vi "Clot.vi"() -> ()   [LabVIEW 2022 SP3]
uses:
  <vilib>/Motion/FlexMotion/CustomControls/CustomControls.llb/AxisOrVectorSpace To Configure.flx
  <vilib>/Motion/FlexMotion/FunctionsVIs/StartStopMotion.llb/Stop Motion (8 axes).flx
panel:
  out "Custom Wave":waveform(i16)(graph)
  out "Actual Time":sgl format="%.2f"
  out "Progress":dbl(slide) scale=0.0..1.0 scale format="%.2f"
  in  "Panametrics":bool
  in  "Temp":bool=TRUE
  in  "Motion Stage Type":u16(ring)=2 items=["MM 2000", "Servo", "Stepper"]
  in  "Digitizer":bool
  in  "Move Motors":bool
  in  "START EXP":bool
  in  "QUIT":bool
  out "Current Pass":i32
  in  "Exp Select":enum32{"PW", "Stop and Go", "F Balance"}(tab)
  out "Length time (s)":sgl=1.0 min=-2e+07 max=2e+07 format="%.2f"
  out "Number of passes":i32
  in  "exp per cycle  (ms)":sgl=0.5 format="%.3f"
  in  "scan length (cm)":sgl=1.0 min=-2e+07 max=2e+07 format="%.2f"
  in  "Total exp time (s)":dbl=10.0 format="%.2f"
  in  "Velocity (cm/s)":sgl=1.0 format="%.2f"
  in  "duty cycle":dbl=0.5 format="%.3f"
  out "PRF (Hz)":dbl=1000.0
  in  "Load Wave?":bool
  in  "2nd Busrt Scale":dbl=0.5
  in  "Mode":bool caption="Boolean"
  in  "Exp time (s)":dbl=0.3 format="%.2f"
  in  "exp per cycle  (ms) sg":sgl=0.5 format="%.3f"
  in  "duty cycle sq":dbl=0.5 caption="duty cycle sg" format="%.3f"
  out "PRF (Hz) sg":dbl=1000.0 caption="PRF (Hz)"
  out "Total exp pts":i16=1
  out "Total one way dist (mm)":sgl=1.0 format="%.2f"
  in  "Number of Repeats":i16=1
  in  "Total exp pts in one direction":i16=2 min=2
  in  "Time for move between exp (s)":sgl=1.0 format="%.2f"
  in  "Dist between exp (mm)":sgl=1.0 format="%.2f"
  in  "On time (s)":dbl=0.3 format="%.2f"
  # "Motion system is initialized on first execution. Wait for motion window to open before turning on motor amplifier. Function generator must be in burst, ext gate mode. The Ext Trig on grey box goes to gate of HP 3352A. Stages return to start position after scan or if scan interupted. TURN OFF ENI BEFORE QUITING LABVIEW!"
  # "Red means off, green means active. Scan can be stopped by switching to red."
  # "Motion may stop mid length if actual time exceeds Total exp time."
  # "Exposure Values"
  # "Motion values"
  # "Exposure Values"
  # "Pressing Start Exp turns on  therapy device for specified on time."
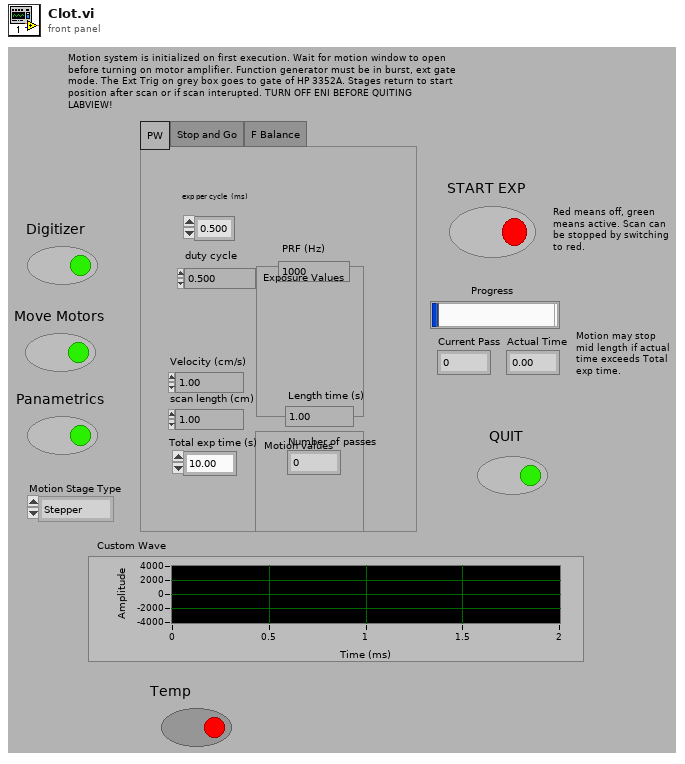
[diagram p1: front panel]
types:
  T1 = typedef "AxisOrVectorSpace To Configure.flx" = u16
  T2 = enum16{"Absolute Position", "Relative Position", "Velocity", "Relative to Cap Pos", "Modulus Position", "Absolute Contouring", "Relative Contouring"}
  T3 = typedef "Resource Out (Enum).flx" = u16
  T4 = typedef "Bd Id Out" = u8
  T5 = cluster{"Reserved":bool, "Axis #1 Move Complete":bool, "Axis #2 Move Complete":bool, "Axis #3 Move Complete":bool, "Axis #4 Move Complete":bool, "Axis #5 Move Complete":bool, "Axis #6 Move Complete":bool, "Axis #7 Move Complete":bool, "Axis #8 Move Complete":bool, "Axis #9 MoveComplete":bool, "Axis #10 Move Complete":bool, "Axis #11 Move Complete":bool, "Axis #12 Move Complete":bool, "Status #13":bool, "Status #14":bool, "Status #15":bool}
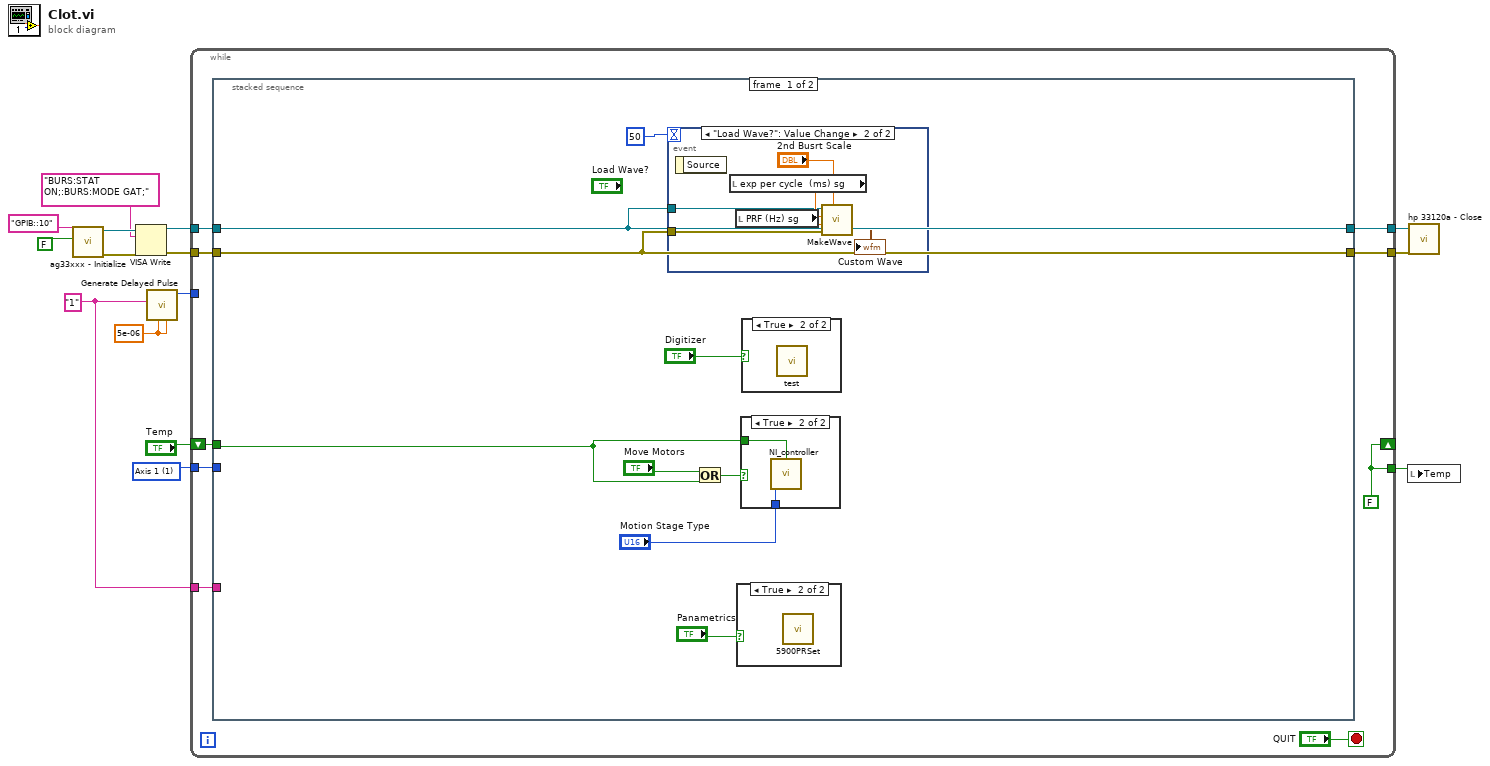
[diagram p0: block diagram]
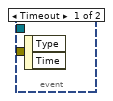
[diagram p2: hidden frame]
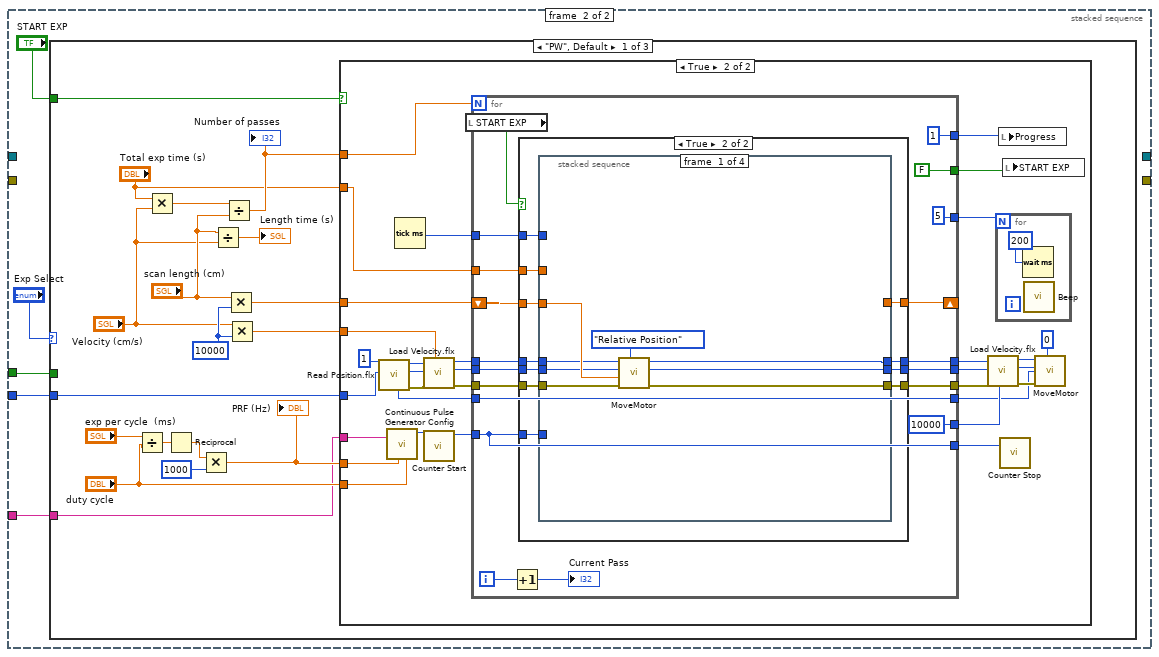
[diagram p6: hidden frame]
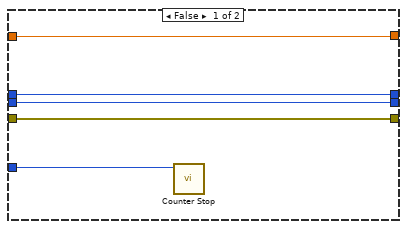
[diagram p8: hidden frame]
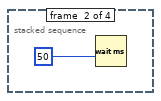
[diagram p9: hidden frame]
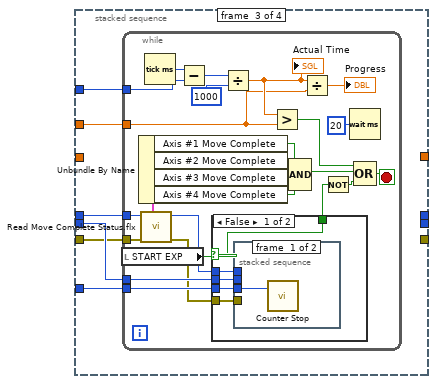
[diagram p10: hidden frame]
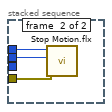
[diagram p11: hidden frame]
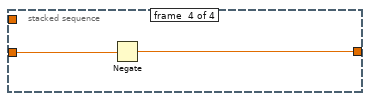
[diagram p13: hidden frame]
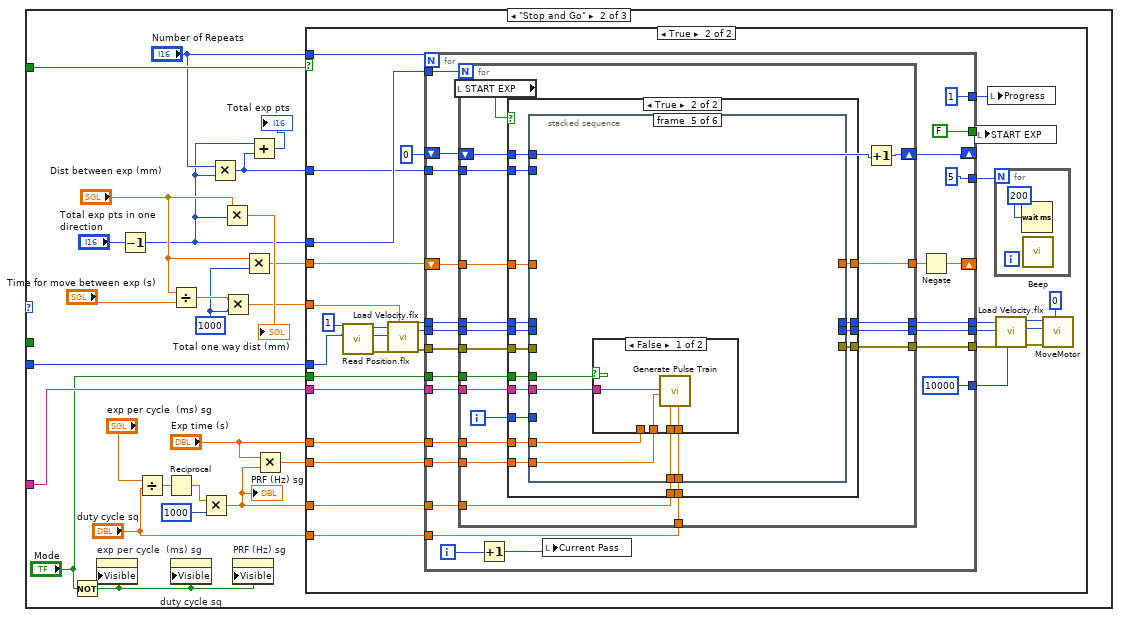
[diagram p14: hidden frame]
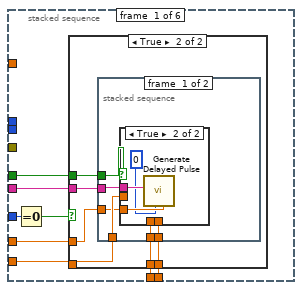
[diagram p17: hidden frame]
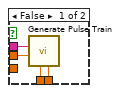
[diagram p19: hidden frame]
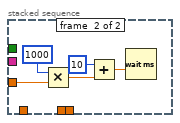
[diagram p20: hidden frame]
diagram:
  w10 = T1 1 items=["Axis 1"=1, "Axis 2"=2, "Axis 3"=3, "Axis 4"=4, "Axis 5"=5, "Axis 6"=6, "Vector Space 1"=17, "Vector Space 2"=18, "Vector Space 3"=19] ("Axis or Vector Space")
  w11 = "1"
  w13 = 5e-06
  n1 = call <instrlib>:"ag33xxx - Initialize.vi"("ID Query (T: Check)"=FALSE, "Instrument Resource Name"="GPIB::10" ("HP33120A Burst")) -> ("error out"=w7:errorcluster, "dup VISA session"=w8:refnum<visa-resource-name>)  [unwired: 8 in]
  n2 = VISA Write(VISA resource name=w8, write buffer="BURS:STAT ON;:BURS:MODE GAT;", error in (no error)=w7) -> (VISA resource name out=w5:refnum<visa-resource-name>, error out=w4:errorcluster)  [unwired: 1 out]
  n3 = call <vilib>:"Generate Delayed Pulse.vi"("pulse width (s or cycles)"=w13, "pulse delay (s or cycles)"=w13, "counter"=w11) -> ("[taskID]"=w12:u32)  [unwired: 6 in, 2 out]
  n4 = while {
    shift-right: [w22] -> _
    shift-left: "Temp" -> [w23]
    tunnel: [w22] -> w14
    tunnel: w12 -> [_]
    tunnel: w11 -> [w21]
    tunnel: w10 -> [w20]
    tunnel: w5 -> [w19]
    tunnel: w4 -> [w18]
    tunnel: [w17] -> w3
    tunnel: [w16] -> w2
    stop <- "QUIT" stop-if-true
    w22 = FALSE
    n5 = stacked-sequence {
      tunnel: w23 -> [w28 w46]
      tunnel: w21 -> [_ w44]
      tunnel: w20 -> [_ w43]
      tunnel: w19 -> [w26 _]
      tunnel: w18 -> [w25 _]
      tunnel: [w26 _] -> w17
      tunnel: [w25 _] -> w16
      frame #0 {
        n6 = event shown="[1] \"Load Wave?\": Value Change" {
          selector: _ -> [_ _]
          dyn-events: _ -> [_ _]
          timeout: 50 -> [_ _]
          tunnel: w26 -> [_ w36]
          tunnel: w25 -> [_ w35]
          event Timeout {
            n7 = event-data() -> ()  [unwired: 1 in, 2 out]
          }
          event "Load Wave?": Value Change {
            n8 = event-data() -> ()  [unwired: 1 in, 1 out]
            n9 = local read "exp per cycle  (ms) sg"() -> (w38:sgl)
            n10 = local read "PRF (Hz) sg"() -> (w39:dbl)
            n11 = call "MakeWave.vi"("Instrument Resource Name"=w36, "exp per cycle  (ms) sg"=w38, "PRF (Hz) sg"=w39, "error in (no error)"=w35, "2nd Busrt Scale"="2nd Busrt Scale") -> ("output waveform"=→"Custom Wave":waveform(i16))  [unwired: 1 out]
          }
        }
        n12 = Or(x="Move Motors", y=w28) -> (x .or. y?=w29:bool)
        n13 = case shown="True" "Panametrics" {
          frame False {
          }
          frame True {
            n14 = call "5900PRSet.vi"() -> ()  [unwired: 13 in, 3 out]
          }
        }
        n15 = case shown="True" w29 {
          tunnel: "Motion Stage Type" -> [_ w41]
          tunnel: w28 -> [_ w40]
          frame False {
          }
          frame True {
            n16 = call "NI_controller.VI"("Initialize"=w40, "Motion System"=w41) -> ()  [unwired: 3 in, 1 out]
          }
        }
        n17 = case shown="True" "Digitizer" {
          frame False {
          }
          frame True {
            n18 = call "test.vi"() -> ()  [unwired: 4 in, 4 out]
          }
        }
      }
      frame #1 {
        n19 = case shown="\"PW\", Default" "Exp Select" {
          tunnel: w46 -> [_ _ _]
          tunnel: w44 -> [w49 w203 w393]
          tunnel: w43 -> [w48 w204 _]
          tunnel: "START EXP" -> [w47 w208 w395]
          frame "PW", Default {
            w64 = 10000
            n20 = Divide(x="exp per cycle  (ms)", y="duty cycle") -> (x/y=w61:dbl)
            n21 = Multiply(x="Total exp time (s)", y="Velocity (cm/s)") -> (x*y=w63:dbl)
            n22 = Reciprocal(x=w61) -> (1/x=w60:dbl)
            n23 = Multiply(x=w60, y=1000) -> (x*y=w55:dbl)
            "PRF (Hz)" <- w55
            n24 = Divide(x="scan length (cm)", y="Velocity (cm/s)") -> (x/y=→"Length time (s)":sgl)
            n25 = Divide(x=w63, y="scan length (cm)") -> (x/y=w56:dbl)
            "Number of passes" <- w56
            n26 = Multiply(x="scan length (cm)", y=w64) -> (x*y=w58:sgl)
            n27 = Multiply(x="Velocity (cm/s)", y=w64) -> (x*y=w57:sgl)
            n28 = case shown="True" w47 {
              tunnel: w58 -> [_ w93]
              tunnel: w57 -> [_ w92]
              tunnel: w56 -> [_ w91]
              tunnel: w55 -> [_ w90]
              tunnel: "duty cycle" -> [_ w89]
              tunnel: "Total exp time (s)" -> [_ w85]
              tunnel: w49 -> [_ w66]
              tunnel: w48 -> [_ w65]
              frame False {
              }
              frame True {
                n29 = call <vilib>:"Read Position.flx"("Axis"=w65, "Board ID"=1) -> ("error out"=w80:errorcluster, "Resource Output"=w79:T3, "Bd ID Out"=w82:T4, "Position"=w72:i32)  [unwired: 4 in]
                n30 = call <vilib>:"Continuous Pulse Generator Config.vi"("duty cycle (0.5)"=w89, "frequency (Hz)"=w90, "counter"=w66) -> ("taskID"=w96:u32)  [unwired: 5 in, 3 out]
                n31 = Tick Count (ms)() -> (millisecond timer value=w84:u32)
                n32 = call <vilib>:"Load Velocity.flx"("Velocity (10000)"=w92, "error in (no error)"=w80, "Axis or Vector Space"=w79, "Board ID"=w82) -> ("error out"=w74:errorcluster, "Resource Output"=w78:T3, "Bd ID Out"=w77:T4)  [unwired: 3 in]
                n33 = call <vilib>:"Counter Start.vi"("taskID"=w96) -> ("taskID"=w95:u32)  [unwired: 9 in, 1 out]
                n34 = for {
                  N: w91 -> [_]
                  shift-right: [w114] -> _
                  shift-left: w93 -> [w116]
                  tunnel: w77 -> [w115]
                  tunnel: w95 -> [w113]
                  tunnel: [w113] -> w94
                  tunnel: [FALSE] -> w86
                  tunnel: [5] -> w88
                  tunnel: [10000] -> w87
                  tunnel: w85 -> [w106]
                  tunnel: w84 -> [w105]
                  tunnel: [1] -> w83
                  tunnel: w78 -> [w103]
                  tunnel: [w102] -> w76
                  tunnel: [w101] -> w75
                  tunnel: w74 -> [w100]
                  tunnel: [w99] -> w73
                  tunnel: [w98] -> w68
                  tunnel: w72 -> [w98]
                  i -> [w111]
                  n35 = local read "START EXP"() -> (w107:bool)
                  n36 = Increment(x=w111) -> (x+1=→"Current Pass":i32)
                  n37 = case shown="True" w107 {
                    tunnel: w116 -> [w120 w132]
                    tunnel: w115 -> [w119 w131]
                    tunnel: [w120 w130] -> w114
                    tunnel: w113 -> [w121 w129]
                    tunnel: w106 -> [_ w128]
                    tunnel: w105 -> [_ w127]
                    tunnel: w103 -> [w118 w126]
                    tunnel: [w119 w125] -> w102
                    tunnel: [w118 w124] -> w101
                    tunnel: w100 -> [w117 w123]
                    tunnel: [w117 w122] -> w99
                    frame False {
                      n38 = call <vilib>:"Counter Stop.vi"("taskID"=w121) -> ()  [unwired: 5 in, 2 out]
                    }
                    frame True {
                      n39 = stacked-sequence {
                        tunnel: w132 -> [w140 _ _ w184]
                        tunnel: w131 -> [w136 _ w147 _]
                        tunnel: [_ _ _ w183] -> w130
                        tunnel: w129 -> [_ _ w146 _]
                        tunnel: w128 -> [_ _ w145 _]
                        tunnel: w127 -> [_ _ w144 _]
                        tunnel: w126 -> [w133 _ w143 _]
                        tunnel: [w135 _ _ _] -> w125
                        tunnel: [w134 _ _ _] -> w124
                        tunnel: w123 -> [w138 _ w142 _]
                        tunnel: [w137 _ _ _] -> w122
                        frame #0 {
                          n40 = call "MoveMotor.vi"("Position Mode (Absolute)"=T2."Relative Position", "error in (no error)"=w138, "Target Position (0)"=w140, "Axis or Vector Space"=w133, "Motion Bd ID"=w136) -> ("error out"=w137:errorcluster, "Resource Output"=w134:u16, "Bd ID Out"=w135:u8)  [unwired: 4 in]
                        }
                        frame #1 {
                          n41 = Wait (ms)(milliseconds to wait=50) -> ()  [unwired: 1 out]
                        }
                        frame #2 {
                          n42 = while {
                            tunnel: w147 -> [w167]
                            tunnel: w146 -> [w165]
                            tunnel: w143 -> [w164]
                            tunnel: w145 -> [w149]
                            tunnel: w144 -> [w155]
                            tunnel: w142 -> [w152]
                            stop <- w161 stop-if-true
                            n43 = local read "START EXP"() -> (w166:bool)
                            n44 = call <vilib>:"Read Move Complete Status.flx"("error in (no error)"=w152, "Board ID"=w167) -> ("error out"=w151:errorcluster, "Bd ID Out"=w153:T4, "Move Complete Status"=w172:T5)  [unwired: 4 in]
                            n45 = Unbundle By Name(w172) -> ("Axis #1 Move Complete"=w171:bool, "Axis #2 Move Complete"=w170:bool, "Axis #3 Move Complete"=w169:bool, "Axis #4 Move Complete"=w168:bool)
                            n46 = Tick Count (ms)() -> (millisecond timer value=w160:u32)
                            n47 = Subtract(x=w160, y=w155) -> (x-y=w159:u32)
                            n48 = case shown="False" w166 {
                              selector: w166 -> [w174 w182]
                              tunnel: w165 -> [w177 _]
                              tunnel: w164 -> [w176 _]
                              tunnel: w153 -> [w175 _]
                              tunnel: [w174 w182] -> w162
                              tunnel: w151 -> [w173 _]
                              frame False {
                                n49 = stacked-sequence {
                                tunnel: w177 -> [w178 _]
                                tunnel: w176 -> [_ w181]
                                tunnel: w175 -> [_ w180]
                                tunnel: w173 -> [_ w179]
                                frame #0 {
                                n50 = call <vilib>:"Counter Stop.vi"("taskID"=w178) -> ()  [unwired: 5 in, 2 out]
                                }
                                frame #1 {
                                n51 = call-poly <vilib>:"Stop Motion.flx"("error in (no error)"=w179, "Axis or Vector Space"=w181, "Board ID"=w180) -> ()  [unwired: 4 in, 3 out]
                                }
                                }
                              }
                              frame True {
                              }
                            }
                            n52 = Divide(x=w159, y=1000) -> (x/y=w150:dbl)
                            "Actual Time" <- w150
                            n53 = Greater?(x=w150, y=w149) -> (0:w148:bool)
                            n54 = Compound Arithmetic op=AND(w171, w170, w169, w168) -> (w163:bool)
                            n55 = Divide(x=w150, y=w149) -> (x/y=→"Progress":dbl)
                            n56 = Not(x=w162) -> (.not. x?=w154:bool)
                            n57 = Wait (ms)(milliseconds to wait=20) -> ()  [unwired: 1 out]
                            n58 = Compound Arithmetic op=OR(w148, w163, w154) -> (w161:bool)
                          }
                        }
                        frame #3 {
                          n59 = Negate(x=w184) -> (-x=w183:sgl)
                        }
                      }
                    }
                  }
                }
                n60 = call <vilib>:"Load Velocity.flx"("Velocity (10000)"=w87, "error in (no error)"=w73, "Axis or Vector Space"=w75, "Board ID"=w76) -> ("error out"=w70:errorcluster, "Resource Output"=w69:T3, "Bd ID Out"=w71:T4)  [unwired: 3 in]
                n61 = for {
                  N: w88 -> [_]
                  n62 = Wait (ms)(milliseconds to wait=200) -> ()  [unwired: 1 out]
                  n63 = call <vilib>:"Beep.vi"() -> ()  [unwired: 12 in]
                }
                n64 = local write "Progress"(w83) -> ()
                n65 = call <vilib>:"Counter Stop.vi"("taskID"=w94) -> ()  [unwired: 5 in, 2 out]
                n66 = local write "START EXP"(w86) -> ()
                n67 = call "MoveMotor.vi"("Position Mode (Absolute)"=0, "error in (no error)"=w70, "Target Position (0)"=w68, "Axis or Vector Space"=w69, "Motion Bd ID"=w71) -> ()  [unwired: 4 in, 3 out]
              }
            }
          }
          frame "Stop and Go" {
            w201 = 1000
            n68 = Not(x="Mode") -> (.not. x?=w188:bool)
            n69 = property on="exp per cycle  (ms) sg" class="DigNum (strict)"("Visible"=w188) -> ()  [unwired: 2 in, 2 out]
            n70 = Decrement(x="Total exp pts in one direction") -> (x-1=w185:i16)
            n71 = Divide(x="exp per cycle  (ms) sg", y="duty cycle sq") -> (x/y=w197:dbl)
            n72 = Reciprocal(x=w197) -> (1/x=w196:dbl)
            n73 = Divide(x="Dist between exp (mm)", y="Time for move between exp (s)") -> (x/y=w206:sgl)
            n74 = property on="duty cycle sq" class="DigNum (strict)"("Visible"=w188) -> ()  [unwired: 2 in, 2 out]
            n75 = Multiply(x=w196, y=1000) -> (x*y=w191:dbl)
            "PRF (Hz) sg" <- w191
            n76 = Multiply(x="Number of Repeats", y=w185) -> (x*y=w187:i16)
            n77 = Multiply(x="Dist between exp (mm)", y=w185) -> (x*y=→"Total one way dist (mm)":sgl)
            n78 = Multiply(x=w206, y=w201) -> (x*y=w205:sgl)
            n79 = property on="PRF (Hz) sg" class="DigNum (strict)"("Visible"=w188) -> ()  [unwired: 2 in, 2 out]
            n80 = Multiply(x="Dist between exp (mm)", y=w201) -> (x*y=w200:sgl)
            n81 = Add(x=w185, y=w187) -> (x+y=→"Total exp pts":i16)
            n82 = Multiply(x="Exp time (s)", y=w191) -> (x*y=w190:dbl)
            n83 = case shown="True" w208 {
              tunnel: w205 -> [_ w232]
              tunnel: w204 -> [_ w231]
              tunnel: w203 -> [_ w222]
              tunnel: "Exp time (s)" -> [_ w221]
              tunnel: "Number of Repeats" -> [_ w220]
              tunnel: w200 -> [_ w219]
              tunnel: w185 -> [_ w216]
              tunnel: w187 -> [_ w215]
              tunnel: "duty cycle sq" -> [_ w213]
              tunnel: w191 -> [_ w212]
              tunnel: w190 -> [_ w211]
              tunnel: "Mode" -> [_ w210]
              frame False {
              }
              frame True {
                n84 = call <vilib>:"Read Position.flx"("Axis"=w231, "Board ID"=1) -> ("error out"=w238:errorcluster, "Resource Output"=w237:T3, "Bd ID Out"=w240:T4)  [unwired: 4 in, 1 out]
                n85 = call <vilib>:"Load Velocity.flx"("Velocity (10000)"=w232, "error in (no error)"=w238, "Axis or Vector Space"=w237, "Board ID"=w240) -> ("error out"=w228:errorcluster, "Resource Output"=w229:T3, "Bd ID Out"=w230:T4)  [unwired: 3 in]
                n86 = for {
                  N: w220 -> [_]
                  shift-right: [w251] -> _
                  shift-left: w219 -> [w265]
                  tunnel: [FALSE] -> w217
                  tunnel: [5] -> w227
                  tunnel: [10000] -> w223
                  tunnel: [1] -> w218
                  tunnel: [w259] -> w226
                  tunnel: [w258] -> w225
                  tunnel: [w257] -> w224
                  tunnel: w230 -> [w256]
                  tunnel: w229 -> [w255]
                  tunnel: w228 -> [w254]
                  tunnel: w222 -> [w253]
                  tunnel: w221 -> [w252]
                  tunnel: w216 -> [w250]
                  tunnel: w215 -> [w249]
                  shift-right: [w247] -> _
                  shift-left: 0 -> [w248]
                  tunnel: w213 -> [w246]
                  tunnel: w212 -> [w245]
                  tunnel: w211 -> [w244]
                  tunnel: w210 -> [w243]
                  i -> [w242]
                  n87 = for {
                    N: w250 -> [_]
                    tunnel: w265 -> [w284]
                    tunnel: [w283] -> w264
                    tunnel: [w281] -> w259
                    tunnel: [w280] -> w258
                    tunnel: [w279] -> w257
                    tunnel: w256 -> [w278]
                    tunnel: w255 -> [w277]
                    tunnel: w254 -> [w276]
                    tunnel: w253 -> [w275]
                    tunnel: w252 -> [w274]
                    tunnel: w249 -> [w272]
                    shift-right: [w271] -> w247
                    shift-left: w248 -> [w270]
                    tunnel: w246 -> [w269]
                    tunnel: w245 -> [w268]
                    tunnel: w244 -> [w267]
                    tunnel: w243 -> [w266]
                    i -> [w273]
                    n88 = local read "START EXP"() -> (w282:bool)
                    n89 = case shown="True" w282 {
                      tunnel: w284 -> [w288 w305]
                      tunnel: [w288 w304] -> w283
                      tunnel: [w287 w303] -> w281
                      tunnel: [w286 w302] -> w280
                      tunnel: [w285 w301] -> w279
                      tunnel: w278 -> [w287 w298]
                      tunnel: w277 -> [w286 w297]
                      tunnel: w276 -> [w285 w296]
                      tunnel: w275 -> [_ w300]
                      tunnel: w274 -> [_ w299]
                      tunnel: w273 -> [_ w295]
                      tunnel: w272 -> [_ w294]
                      tunnel: w270 -> [_ w293]
                      tunnel: w269 -> [_ w292]
                      tunnel: w268 -> [_ w291]
                      tunnel: w267 -> [_ w290]
                      tunnel: w266 -> [_ w289]
                      frame False {
                      }
                      frame True {
                        n90 = stacked-sequence {
                          tunnel: w305 -> [_ w345 _ _ _ w391]
                          tunnel: [_ _ _ _ _ w391] -> w304
                          tunnel: [_ w342 _ _ _ _] -> w303
                          tunnel: [_ w341 _ _ _ _] -> w302
                          tunnel: [_ w343 _ _ _ _] -> w301
                          tunnel: w300 -> [w313 _ _ _ w375 _]
                          tunnel: w299 -> [w312 _ _ _ w373 w386]
                          tunnel: w298 -> [_ w340 _ w350 _ _]
                          tunnel: w297 -> [_ w339 _ _ _ _]
                          tunnel: w296 -> [_ w338 _ w349 _ _]
                          tunnel: w295 -> [w311 _ _ _ _ _]
                          tunnel: w294 -> [_ _ _ w348 _ _]
                          tunnel: w293 -> [_ _ _ w347 _ _]
                          tunnel: w292 -> [w309 _ _ _ w378 _]
                          tunnel: w291 -> [w308 _ _ _ w377 _]
                          tunnel: w290 -> [w307 _ _ _ w376 _]
                          tunnel: w289 -> [w306 _ _ _ w374 _]
                          frame #0 {
                            n91 = Equal To 0?(x=w311) -> (x = 0?=w310:bool)
                            n92 = case shown="True" w310 {
                              tunnel: w313 -> [_ w319]
                              tunnel: w312 -> [_ w315]
                              tunnel: w309 -> [_ w318]
                              tunnel: w308 -> [_ w317]
                              tunnel: w307 -> [_ w316]
                              tunnel: w306 -> [_ w314]
                              frame False {
                              }
                              frame True {
                                n93 = stacked-sequence {
                                tunnel: w319 -> [w323 _]
                                tunnel: w318 -> [w325 _]
                                tunnel: w317 -> [w324 _]
                                tunnel: w316 -> [w322 _]
                                tunnel: w315 -> [w320 w333]
                                tunnel: w314 -> [w321 _]
                                frame #0 {
                                n94 = case shown="True" w321 {
                                tunnel: w325 -> [w329 _]
                                tunnel: w324 -> [w328 _]
                                tunnel: w323 -> [w327 w332]
                                tunnel: w322 -> [w326 _]
                                tunnel: w320 -> [_ w331]
                                frame False {
                                n95 = call <vilib>:"Generate Pulse Train.vi"("duty cycle (0.5)"=w329, "frequency (Hz)"=w328, "number of pulses (cont:0)"=w326, "counter"=w327) -> ()  [unwired: 5 in, 3 out]
                                }
                                frame True {
                                n96 = call <vilib>:"Generate Delayed Pulse.vi"("pulse width (s or cycles)"=w331, "pulse delay (s or cycles)"=0, "counter"=w332) -> ()  [unwired: 6 in, 3 out]
                                }
                                }
                                }
                                frame #1 {
                                n97 = Multiply(x=1000, y=w333) -> (x*y=w335:dbl)
                                n98 = Add(x=10, y=w335) -> (x+y=w336:dbl)
                                n99 = Wait (ms)(milliseconds to wait=w336) -> ()  [unwired: 1 out]
                                }
                                }
                              }
                            }
                          }
                          frame #1 {
                            n100 = call "MoveMotor.vi"("Position Mode (Absolute)"=T2."Relative Position", "error in (no error)"=w338, "Target Position (0)"=w345, "Axis or Vector Space"=w339, "Motion Bd ID"=w340) -> ("error out"=w343:errorcluster, "Resource Output"=w341:u16, "Bd ID Out"=w342:u8)  [unwired: 4 in]
                          }
                          frame #2 {
                            n101 = Wait (ms)(milliseconds to wait=50) -> ()  [unwired: 1 out]
                          }
                          frame #3 {
                            n102 = while {
                              tunnel: w350 -> [w354]
                              tunnel: w349 -> [w353]
                              tunnel: w348 -> [w352]
                              tunnel: w347 -> [w351]
                              stop <- w360 stop-if-true
                              n103 = local read "START EXP"() -> (w363:bool)
                              n104 = call <vilib>:"Read Move Complete Status.flx"("error in (no error)"=w353, "Board ID"=w354) -> ("error out"=w356:errorcluster, "Bd ID Out"=w357:T4, "Move Complete Status"=w368:T5)  [unwired: 4 in]
                              n105 = Unbundle By Name(w368) -> ("Axis #1 Move Complete"=w367:bool, "Axis #2 Move Complete"=w366:bool, "Axis #3 Move Complete"=w365:bool, "Axis #4 Move Complete"=w364:bool)
                              n106 = case shown="False" w363 {
                                selector: w363 -> [w370 w372]
                                tunnel: w357 -> [w371 _]
                                tunnel: [w370 w372] -> w361
                                tunnel: w356 -> [w369 _]
                                frame False {
                                n107 = call-poly <vilib>:"Stop Motion.flx"("error in (no error)"=w369, "Board ID"=w371) -> ()  [unwired: 5 in, 3 out]
                                }
                                frame True {
                                }
                              }
                              n108 = Divide(x=w351, y=w352) -> (x/y=w355:dbl)
                              n109 = local write "Progress"(w355) -> ()
                              n110 = Compound Arithmetic op=AND(w367, w366, w365, w364) -> (w362:bool)
                              n111 = Not(x=w361) -> (.not. x?=w358:bool)
                              n112 = Wait (ms)(milliseconds to wait=20) -> ()  [unwired: 1 out]
                              n113 = Compound Arithmetic op=OR(w362, w358) -> (w360:bool)
                            }
                          }
                          frame #4 {
                            n114 = case shown="False" w374 {
                              tunnel: w378 -> [w382 _]
                              tunnel: w377 -> [w381 _]
                              tunnel: w376 -> [w380 _]
                              tunnel: w375 -> [w379 w385]
                              tunnel: w373 -> [_ w384]
                              frame False {
                                n115 = call <vilib>:"Generate Pulse Train.vi"("duty cycle (0.5)"=w382, "frequency (Hz)"=w381, "number of pulses (cont:0)"=w380, "counter"=w379) -> ()  [unwired: 5 in, 3 out]
                              }
                              frame True {
                                n116 = call <vilib>:"Generate Delayed Pulse.vi"("pulse width (s or cycles)"=w384, "pulse delay (s or cycles)"=0, "counter"=w385) -> ()  [unwired: 6 in, 3 out]
                              }
                            }
                          }
                          frame #5 {
                            n117 = Multiply(x=1000, y=w386) -> (x*y=w388:dbl)
                            n118 = Add(x=10, y=w388) -> (x+y=w389:dbl)
                            n119 = Wait (ms)(milliseconds to wait=w389) -> ()  [unwired: 1 out]
                          }
                        }
                      }
                    }
                    n120 = Increment(x=w270) -> (x+1=w271:i32)
                  }
                  n121 = Increment(x=w242) -> (x+1=w241:i32)
                  n122 = local write "Current Pass"(w241) -> ()
                  n123 = Negate(x=w264) -> (-x=w251:sgl)
                }
                n124 = local write "START EXP"(w217) -> ()
                n125 = local write "Progress"(w218) -> ()
                n126 = for {
                  N: w227 -> [_]
                  n127 = Wait (ms)(milliseconds to wait=200) -> ()  [unwired: 1 out]
                  n128 = call <vilib>:"Beep.vi"() -> ()  [unwired: 12 in]
                }
                n129 = call <vilib>:"Load Velocity.flx"("Velocity (10000)"=w223, "error in (no error)"=w224, "Axis or Vector Space"=w225, "Board ID"=w226) -> ("error out"=w235:errorcluster, "Resource Output"=w234:T3, "Bd ID Out"=w236:T4)  [unwired: 3 in]
                n130 = call "MoveMotor.vi"("Position Mode (Absolute)"=0, "error in (no error)"=w235, "Axis or Vector Space"=w234, "Motion Bd ID"=w236) -> ()  [unwired: 5 in, 3 out]
              }
            }
          }
          frame "F Balance" {
            n131 = case shown="True" w395 {
              tunnel: "On time (s)" -> [_ w399]
              tunnel: w393 -> [_ w407]
              frame False {
              }
              frame True {
                n132 = call <vilib>:"Delayed Pulse Generator Config.vi"("pulse width (s or cycles)"=w399, "pulse delay (s or cycles)"=0, "counter"=w407) -> ("error out"=w402:errorcluster, "taskID"=w401:u32)  [unwired: 5 in, 2 out]
                n133 = call <vilib>:"Counter Start.vi"("error in (no error)"=w402, "taskID"=w401) -> ("taskID"=w400:u32)  [unwired: 8 in, 1 out]
                n134 = Add(x=w399, y=0.1) -> (x+y=w398:dbl)
                n135 = Tick Count (ms)() -> (millisecond timer value=w406:u32)
                n136 = while {
                  tunnel: w406 -> [w418]
                  tunnel: w398 -> [w416]
                  tunnel: w400 -> [w411]
                  tunnel: [FALSE] -> w405
                  tunnel: [w409] -> w404
                  tunnel: [w411] -> w403
                  stop <- w409 stop-if-true
                  n137 = local read "START EXP"() -> (w410:bool)
                  n138 = Tick Count (ms)() -> (millisecond timer value=w419:u32)
                  n139 = Subtract(x=w419, y=w418) -> (x-y=w420:u32)
                  n140 = Wait (ms)(milliseconds to wait=20) -> ()  [unwired: 1 out]
                  n141 = Not(x=w410) -> (.not. x?=w414:bool)
                  n142 = Divide(x=w420, y=1000) -> (x/y=w417:dbl)
                  n143 = Greater?(x=w417, y=w416) -> (0:w415:bool)
                  n144 = Or(x=w415, y=w414) -> (x .or. y?=w409:bool)
                }
                n145 = local write "START EXP"(w405) -> ()
                n146 = case shown="True" w404 {
                  tunnel: w403 -> [_ w408]
                  frame False {
                  }
                  frame True {
                    n147 = call <vilib>:"Counter Stop.vi"("taskID"=w408) -> ()  [unwired: 5 in, 2 out]
                  }
                }
              }
            }
          }
        }
      }
    }
  }
  n148 = local write "Temp"(w14) -> ()
  n149 = call <instrlib>:"hp 33120a - Close.vi"("error in (no error)"=w2, "VISA session"=w3) -> ()  [unwired: 1 out]
